vi "day4.vi"() -> ()   [LabVIEW 2025]
panel:
  out "Array 4":string[][](array[string])
  out "Array 3":i16[][](array[numeric])
  out "sum":i16
  out "size(s)":i32[](array[numeric])
  out "Array 2":i16[](array[numeric])
  out "x < y?":bool
  out "Array":string[][](array[string])
  out "subarray":string[][](array[string])
  out "appended array":string[][](array[string])
  in  "s":bool
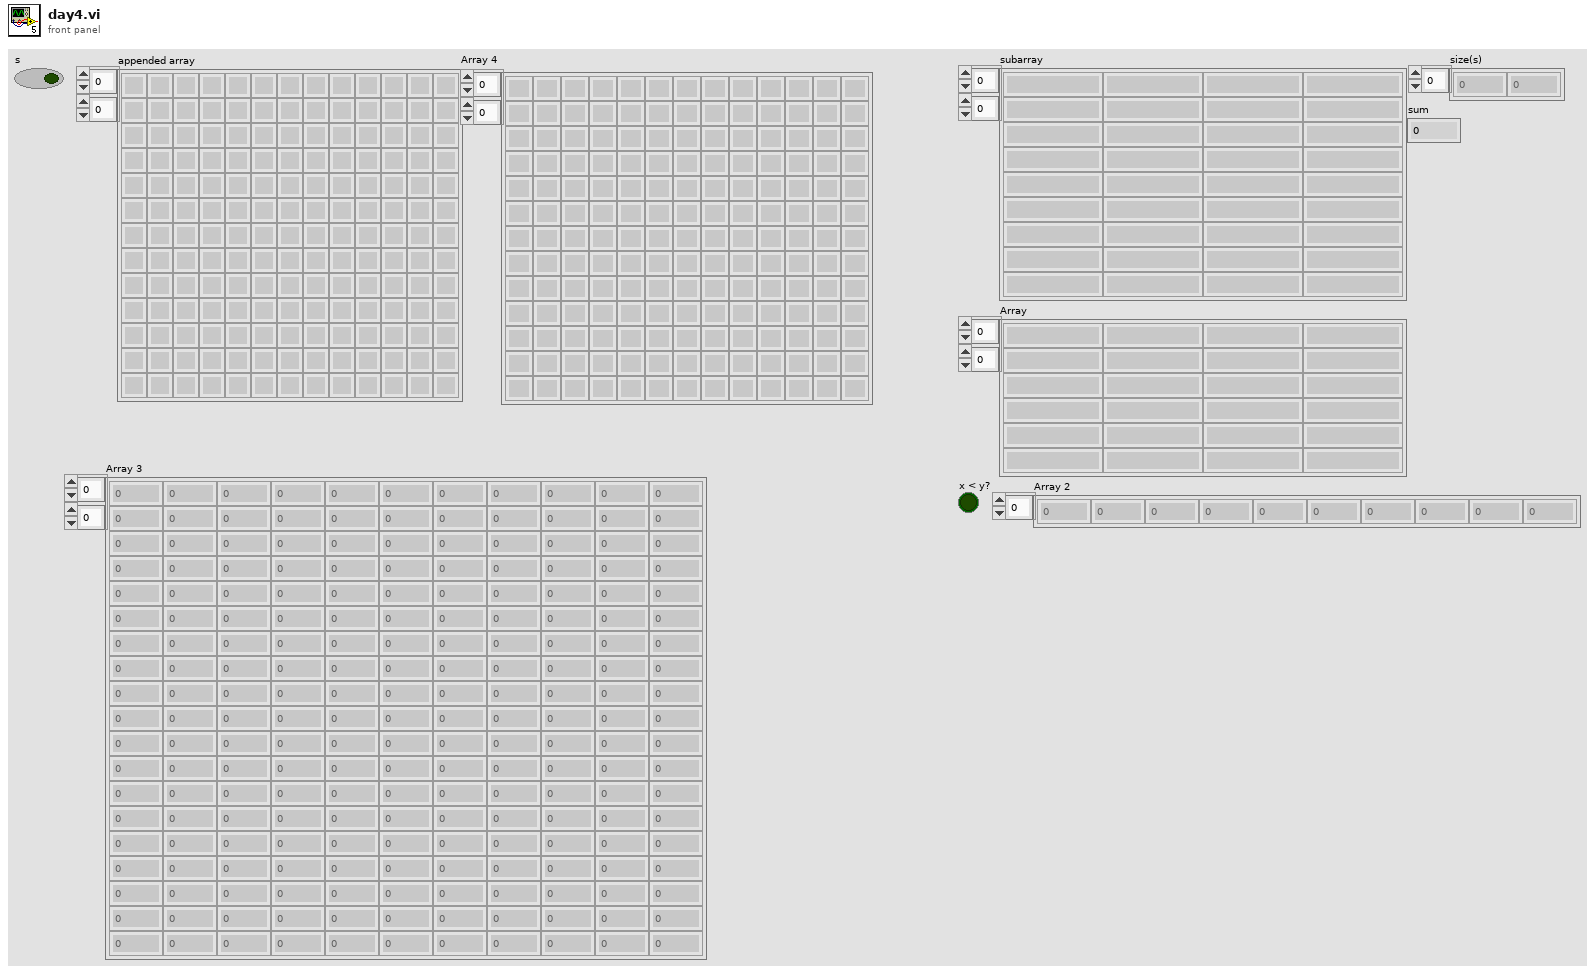
[diagram p1: front panel]
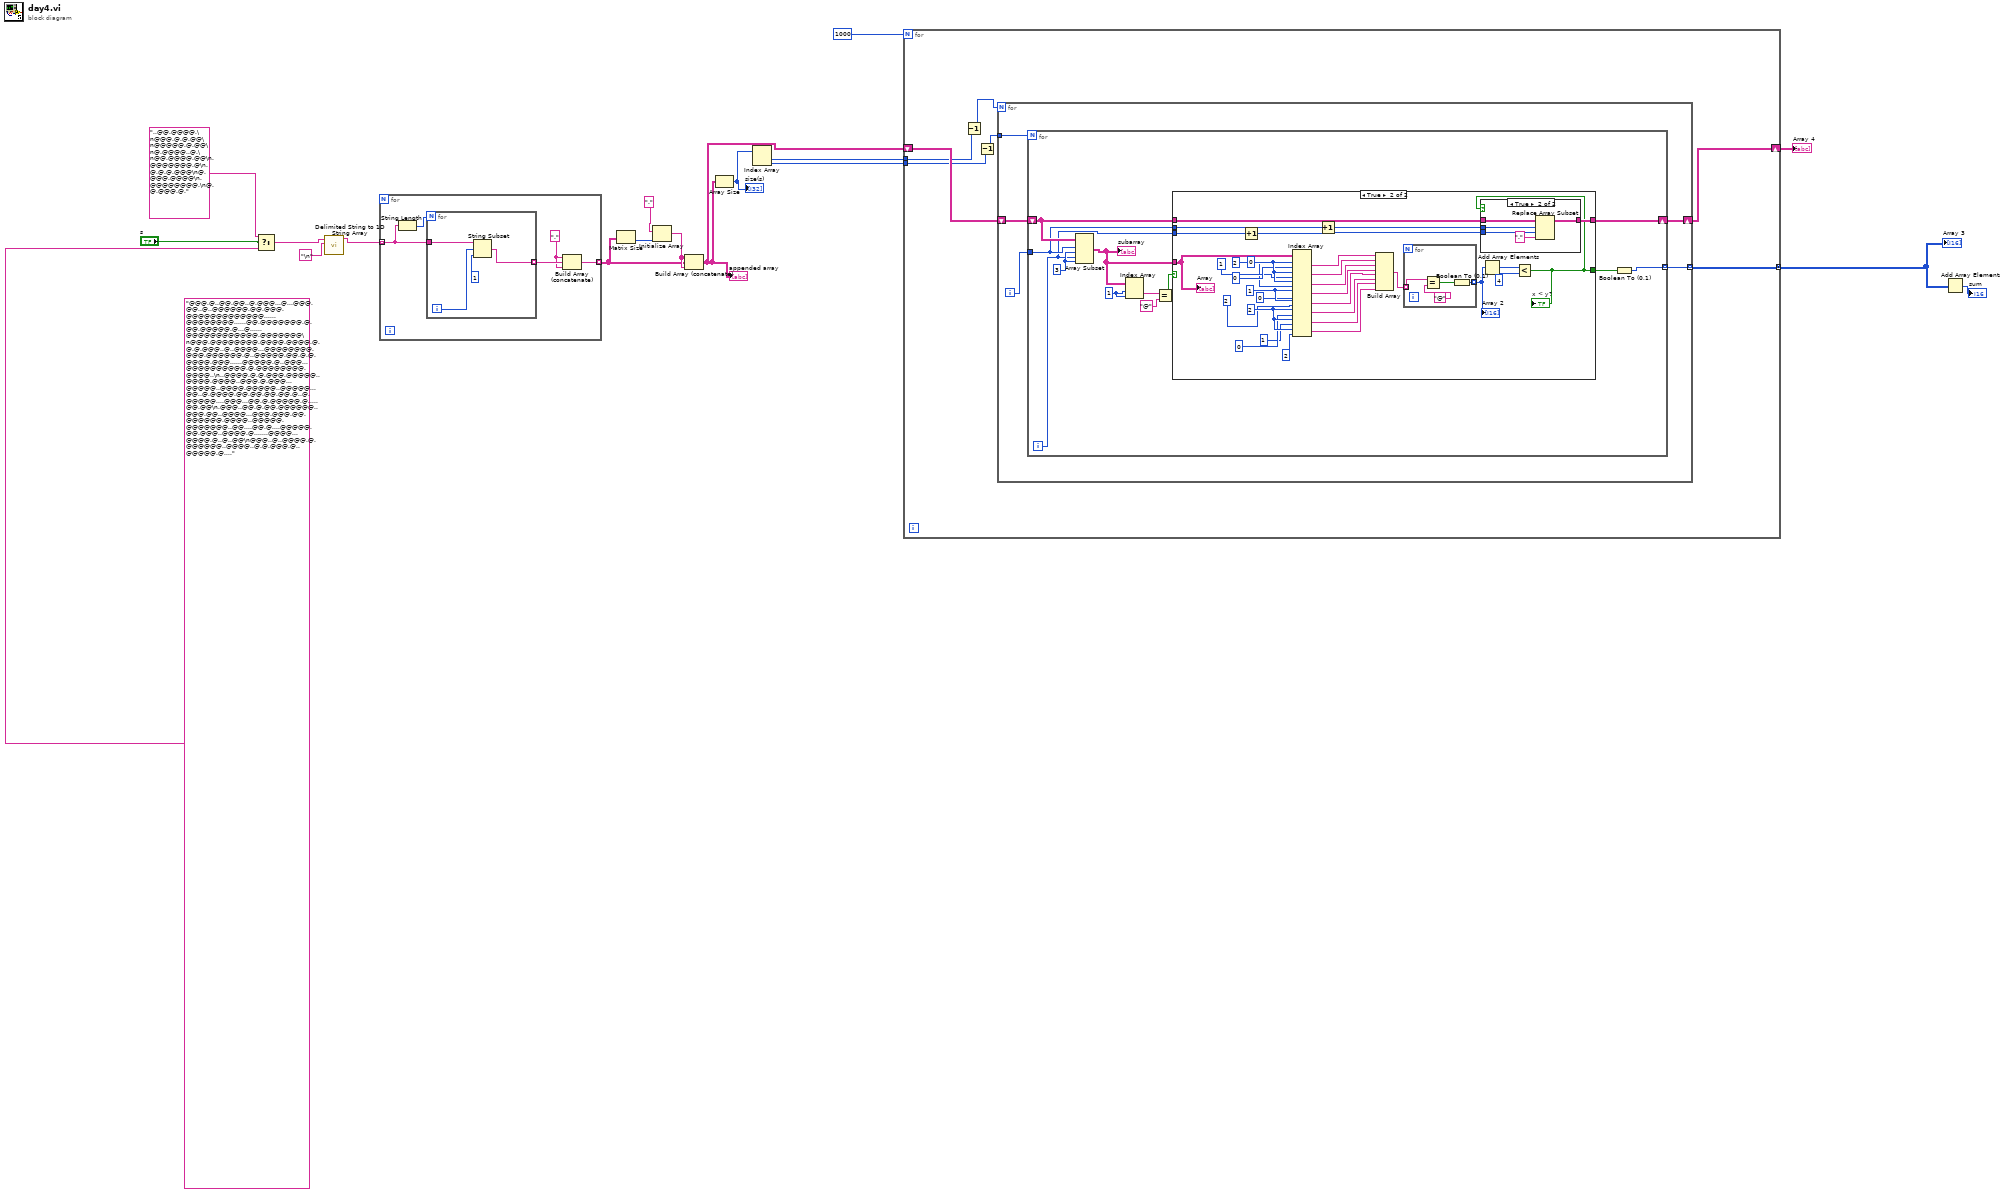
[diagram p0: block diagram]
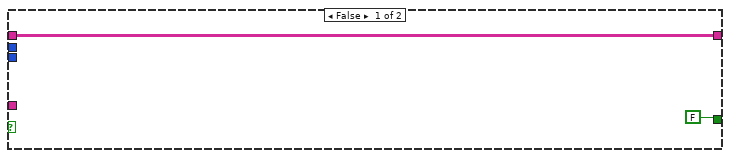
[diagram p2: hidden frame]
diagram:
  n1 = Select(t="..@@.@@@@.\n@@@.@.@.@@\n@@@@@.@.@@\n@.@@@@..@.\n@@.@@@@.@@\n.@@@@@@@.@\n.@.@.@.@@@\n@.@@@.@@@@\n.@@@@@@@@.\n@.@.@@@.@.", s="s", f="@@@.@..@@.@@..@.@@@...@...@@@.@@..@..@@@@@@.@@.@@@.@@@@@@@@@@@@@......@@@@@@@@......@@.@@@@@@@.@.@@.@@@@@.@...@......@@@@@@@@@@@@.@@@@@@@\n@@@.@@@@@@@@.@@@@.@@@@.@.@.@.@@@..@..@@@@...@@@@@@@@.@@@.@@@@@@.@..@@@@@.@@.@.@.@@@@.@@@......@@@@@.@..@@@...@@@@@@@@@@.@.@@@@@@@@.@@@@..\n..@@@@.@.@.@@@.@@@@@..@@@@.@@@@..@@@.@.@@@...@@@@@..@@@@.@@@@@..@@@@@...@@..@.@@@@.@@.@@.@@.@@.@..@.@@@@@....@@@...@@.@.@@@@@.@.....@@.@@\n.@@@..@@.@.@@.@@@@@@..@@@.@@..@@@@...@@@.@@@.@@.@@@@@@.@@@@..@@@@@.@@@@@@@..@@....@@.@....@@@@@.@@.@@@..@@@@.@.......@@@@...@@@@.@..@..@@\n@@@..@..@@@@.@.@@@@@@..@@@@..@.@.@@@.@..@@@@@.@...@..@..@...@....@@..@@@...@@@@@.@.@........@..@@.@.@@...@@@@@.@@@@..@.@@@@...@..@@.@@..@\n@.@@.@.@..@@@@.@.@@@...@@@..@.@.@@..@.@@@......@..@...@.@@.@@@.@@@.@@@@..@@.@.@@@@.@..@..@.@@..@@@@.@@@@@@@@@@@@..@@@@..@@.@.@@..@@..@..@\n.@...@@......@..@@@@@...@@@@@.@@@.@@@@@.@@..@@@@@@@.@@@@@@@@@.@.@..@@@@...@@.@...@@@@@.@@@@@...@.@.@.@@.@@.@.@@.@@@@.@@@@@@@@@.@.@.@...@.\n.@@@...@@@.@....@@@@@@@.@@@.@@@@.@@...@@.@@@@@@...@@@@@..@.@...@.@@..@@..@@@@@@.@@@@@@@@@@..@.@@..@..@.@@..@@.@@@@@@@@...@....@.@@@@@@@@@\n.@..@@@@@@@@.@@@.@@@@@@@.@@@@@.@.@.@@@@..@..@@@..@@@.@@@@.@@.@@@@@..@@@.....@@@.@.@@@@.@@.@.@@@@.@@...@.@@@.@@@@@@@@@..@.@..@@@@@@@.@@@@@\n.@.@@.@.@@@@@@@@@@@..@@@@@@....@@@.@.@.@@@.@@@@@@@@.@@@@@@@..@@..@@@..@@@...@.@@@@..@@@@..@@@@@@@@@@@@.@@.@@@@@@@@@@..@.@.@.@@.@@.@....@.\n@@.@@@@@..@.@.@@@@@@..@@@.@@.@.@@..@@@@.@@..@@@@@@@@.@@@@@@@.@@@@@@@.@@@@...@@@@.@@@@@@@.@@..@@.@.@@@@@.@@@@@@@.@@@@@@@@.@.@.@.@@@@@@@@.@\n..@@.@..@@.@..@.@.@.@@...@@@...@.........@@.@.@@@.@.@@.@.@@.@@@@@@@@.@.@.@@.@@.@@@@@@@@.@@..@@@@@.@@.@@@@@@.@.@.@@@.@.@.@.@@@.@@.@@...@@@\n.@@.@@@..@..@@@....@@@.@@@@@@@@..@@@@..@@.@@@@@..@@.@..@@@@@@@.@@@@@.@@@@.@@@@@@@@@@@.@..@@@..@@.@.@@....@@..@@.@@...@..@@@@@@@..@.@@@@@@\n.@@.@@@@@@.@@@@.@.@.@..@@@@.@..@@..@.@@@@@.@.@@@@@@@@@.@@@..@.@.@.@.@@@@@@@@@@@@...@@.@@@@@@@..@.@.@@@..@...@...@@@@.@@.@@@.@.@.@@@...@..\n@@.@..@@..@@..@.@@@.@@@@.@@@@@@@..@.@@.@@@.@.@.@@@@@@.@@@.@.@@@@@@.@@.@@@.@@@@@@@@@@@@@@@.@.@@@@@@..@@@@..@@.@@.@@@@@.@.@@@@@.@@@@.@@@@@.\n@@@@@.@.@@@.@@..@@.@.@@@@@.@@@..@@@@@@..@...@....@.@@..@@@@.@@@@.@..@@.@@.@@@@.@..@@.@@@@..@@@@.@.@@..@@@@.@.@.@.@@@.@@@@@@.@@@@.@...@@@@\n@@.@@@..@..@.@.@@@@@@@@@@@....@@@@@@@.@.@@@....@@.@@@@@@@@@@..@@.@@.@.@.@..@@.@.@.@...@@.@.@@@@.@@@@@@@@@@@...@.@..@.@..@@@.@@@.@..@@@@..\n.@..@@@..@@.@@.@..@@@@@@..@@@@.@@@@@@@@@@@@.@.@.@@@@@@.@@.@@@@.@@@.@..@@@@@.@@@@@.@.@.@@@@@@.@.@@.@.@.@@@@.@..@@@.@@.@@@.@@.@@@@..@...@@@\n@@....@@.@.@@....@.@@.@@@@@@@@@@@@@..@.@..@@@@.@@.@.@@.@.@@..@..@@@@@@@@@@@@@@@@@@..@.@@@@@@.@..@@@@@.@.....@@@..@...@@@@..@@@@.@@.@@.@@@\n.@...@@@.@@.@.@@.@@@@.@@@@....@@@@@.@@@@@@@@.@@.@@..@@@@.@@.@@@@@.@.@.@@.@.@@@@.@.@@.@@@@..@@@@@@.@@@@.@@.@@..@@@@....@@@@@@.@@.@@@@@@@.@\n.@@.@@@@@@@.@@@.@@.@..@@@.@@@@@@@.@@@@..@@@@@@...@@@..@..@@@@@@@.@@@@...@@@@@..@@@@@@..@@.@@.@@.@@@@@@@@@.@@@@@.@@...@@@@@@@.@@..@.@.@@@.\n@@@@@.@@.@@@.@@@@@@@@@@@@.@.@.@@@@.@@.@...@@@@@@...@@..@@@@.@@@@@@@.@.@@.@@@.@...@.@.@@.@@.@@..@@@@...@@.@@@@.@@@@@@@.@@@..@.@...@@@@@...\n..@@@@@@.@.....@.@..@@.@@@.@@@@.@@@@..@..@.@@....@@@@@.@..@@..@@..@.@@.@@@..@...@@..@@.@@@@@.....@@@@@@@@@@@@..@@@@@@@..@@@.@@.@@.....@@.\n@@@@@.@@.@@.@@.@@@@@@.@@.....@.@..@..@@@@@@.@@@.@@@@@@..@@..@@@.@@@@@.@@@...@..@@@...@@@@.@..@@@@@...@@..@.@@@..@.@@..@@@@.@.@.@@@...@.@@\n@@@@@@@@@@@..@@@@.@@@..@@.@.@@@@@@@.@@..@..@@@....@@@@@..@.@..@@@@@@...@@..@@@@@@@@@@@.@..@..@@@....@.@@@..@@@@..@@....@.@.@@@..@.@.....@\n@.@@.@....@..@@@@@@@@@@@.@........@.@@@@@@@@..@..@.@@.@.@@.@@@..@..@..@...@@@@@@@@.@..@@@...@@@@@@@@.....@@@..@@@.@@@.@@.@@..@.@@.@@@@@@.\n.@@@..@@@@..@@.@.@@@..@.@@.@@@@@@@@@@.@@...@@@@@@@@@...@@..@@.@@..@@@@@.@@@@..@.@..@.@@@.@@.@@@.@@@@.@@@@@@.@@.@@@.@@..@.@@@.@.@@@@@.@@@.\n@@@.@@.@@.@..@..@....@.@@@@@@@..@@.@@@..@@@@@..@@@@@...@...@@@@.@@@.@..@@@..@..@@@@@.@@.@@@@@@.@@@@@.@@@@..@..@@@.@@@@.@@...@..@.@..@@@.@\n@..@.@.@@@.@@@@.@.@@@.@.@@@@..@@@@.@@...@@@....@@..@@.@@@@@@@@.@.@@@@@..@@@@@@@@...@.@.@@@.@@.@...@@@@@.@@....@@.@@@@@@....@.@.@@@@.@.@@.\n@@@@@@..@@..@.@.@...@@@..@....@..@@..@@@@@@@@..@.@...@@@@@@@.@.@@.@@@.@...@@.@@@@@..@@@@@@..@@@@@.@@@.@@@@@@.@@...@@@@@.@.@.@@@@..@.@@..@\n@...@@@@@@@@@@@@.@@@@@@@..@..@.@@@@@..@@@..@@...@..@@.@.@.@@@.......@@@@@....@...@@@@@@@@@@@.@.@.@.@@@@@@.@@@.@@....@@@.@....@@@@@@@@.@@.\n@@.@@@.@@.@.@@@@.@.@.@@@.@.@@@@..@.@@@@@@@@@.@.@@@@.@@@..@...@@@.@.@.@.@@@@@@.@@@@@.@@@..@@@@.@.@@@@@@.@@@@@.@@..@@@@@@@@@@.@..@@@@@@@@@@\n@@.@..@@@@@.@@@@.@@@@@@@@@@@@...@@@@@.@..@..@.@@@@@@@@..@.@@@@@..@.@@@@.@..@@..@@@@@@@@@@..@@@.@.@@@@@@.@@@@.@@@@@@@@@@@@@.@@@@..@@@@@@@@\n.@.@@@@..@.@.@...@@@@.@..@@@@@@@@@...@@@..@.@@@..@@@@@@@@@...@@@@@@.@@@.@@.@@@@@..@@..@@....@@@@@@@@.@@@@.@@..@@@@@@.@.@@@@@.@@@@@.@@@@@.\n.@@@@@@@@@..@..@@@@.@.@.@@@@.@@@...@@.....@.@.@@@@@@@@@@@@@@@@.@.@..@@.@.@@@..@@..@@@@@@@.@@.@@@.@@@@@..@@.@@@@@@@@@@@@..@@@@.@.@.@.@@@@@\n@@.....@.@@@@@@.@@.@@@@@@@@@@@@.@@@@@@.@@@@@@@@...@@..@@.@@.@@@@@@@.@@@.@.@@@...@@@@@@@@.@@@@@@.@@@@.@@@@@@@@.@@..@..@..@@@....@.@@@@.@@.\n@....@..@.@..@.@@@@@@.@.@.@@@@..@.@@@...@@@.@..@.@@@@...@@@@@@@.@.@.@.@@@@@@@@@@@..@.@@..@@.@@@@@@@@...@@@.@@..@.....@@@@@@@@@@..@@.@@.@@\n..@@@...@.@@.@@@.@@@...@..@@@@@.@..@@.@.@@@.@@@.@@..@@@@@@@@@@@@@.@@@@@..@.@.@@@@@@..@@@@..@@@...@.@@@@....@...@@..@@@..@@@@@..@..@.@@...\n.@@@@@@@@.@.@@.@@.@@@@@.@@.@........@@..@@@.@.@@..@@..@@@@.@@@@@.@@.@@@@@@@.@@@.@@@..@@....@@...@@@.@.@.@@@@@@@@.@@@...@@@@@@@@@@.@..@@..\n@.@@.@.@@@@.@.@.@@@@@..@.@.@...@@@.@.@.@.@@@@@@@.@.@@.@@@.@@@@@.@@@@@@.@.@@..@@@..@.@@.@@..@.@@@@@@@@@@.@....@@@.@@@@@@@@@@@@@@@...@@@@..\n@@.@@@..@.@@...@@.@@@@.@@@@@.@.@@.@@@@@@@@@...@@@@@.@@@@@@..@.@@..@@@.@.@@@..@@.....@.@@.@.@.@..@..@@@.@.@@.@@@@@@@.@.@@....@@.@@@@...@@@\n@.@@.@@@@@..@@@@.@..@..@@.@.@.@...@@.........@@.@.@@@@.@@..@@.@@.@@@.@.@.@@.@@.@@..@.@@.@.@@@@@@@@@@@..@.@@@.@@.@@@@@@@.@.@@...@..@@@...@\n@.@@@...@@.@@.@@@@.@@..@@@.@@.@@......@@.@@@..@@.@@..@@@@@.@.@.@@....@..@@@..@@.@@.@@@@@@@.@@@@@@@@...@@@@@@@@@@@@@@@...@...@..@@.@.@@@@@\n@@@@.@@.@@@@@@@@@.@.@@....@...@@.@..@.@.....@@@.@@....@@..@@..@.@.@@@@....@.@@@@@@.@@..@@.@@@.@@@.@@@@@@@@@@@..@.@@..@.@.@@@@@@.@@@@@@.@@\n...@@..@..@@@..@.@@@@@@@.@.@@@.@.@@@.@.@@@.@@.@@@@@..@@.@...@@@..@.@@@@@@@.@.@@@.@@@@@.@@@@@@@@.@@.@.@@@@@.@..@.@@@@@@@@@@.@@...@.@...@@.\n.@@@@@@@@@@..@@@@.@@.@.@@@.@@.@@..@@@.@@@@@.@.@@@..@@@@@@@.@@@@@..@@@@@.@@.@@@..@@@@@.@@@.@..@..@...@.@.@.@@.@@.@@@@@@@.@@@@@.@@.@@@@..@@\n@..@.@.@@..@.@@@@@.@.@@.@..@@@.@@@@..@..@@@@@..@@..@@@@..@.@@.@@.@@@@@@@@@@@@@@......@...@.@@@@.@..@.@.@@...@@@@@@@.@.@@.@@.@@@....@.@@@@\n@@@@@@@@@@.@@@..@@.@@@.@@.@..@@.@@.@@@@@@...@..@.@....@.@@.@@@@@@.@@.@@@.@@.@@@@@......@@.@@..@@@.@.....@@@@@@@@.@@..@@.@.@.@@..@@.@....@\n@@.@@@..@@@.@@@@@@@@@@...@@.@.@.@@.@@.@.@....@@@.@@..@....@.@@.@..@@@.@@@.@..@.@..@..@@@@@@@@@.@.@.@.@...@@@@.@.@@@.@...@@@@@@..@@...@@@@\n@@@@.@@.@@@.@@@@@@@@@@@...@@.@@..@.@@@...@@.@.@.@@@@@@.@@@@..@@@@..@@..@.@.@@@@@.@.@@@@.@@@.@@@.@.@@@..@@.@@..@.@@@@@@@.@@@..@@@@.@.@@@@@\n@...@@.@@@@@@.@.@@@@@@@@@@@@@@@@@@..@@..@@...@@.@.@@@@.@@.@@@@@@@.@.@.@@.@@.@..@.@@@@..@@@...@@.@.@@..@@@....@@.@..@...@.@@@.@@@@@@@...@@\n@@..@..@.@.@@@@.@@@..@.@@@@@@@@.@@@.@@@.@@@.@@..@@.@@@@.@..@.@..@...@@.@@@@...@@@@@..@@@..@...@.@@.@@@.@.@@@.@.@....@..@.@@@@@@@@.@@.@@@@\n@@@@@@..@@@....@@.@.@...@@@@@.@..@@@@@@..@...@@.@@@@@@.@.@@.@@@@.@.@.@@@@@@.@.@@@@@@@@.@...@@@@@@.@.....@@...@@...@@@@@@@.@@@@@@@@.@.@@..\n@@@@@@@@...@@@@..@..@..@@@..@@.@@@@@@.@@@..@@@@.@@.@..@..@.@@.....@.@@..@@@....@@@@@@.@@@@@@@@@@@@..@.@@@@@@@@....@.@@@.@@@@@@@@@@@..@.@.\n@@@@@.@..@.@@.@@@@..@.....@.@@@.@.@.@@@.@@@@@..@@.@@@@@@..@@.@.@@@...@@.@.@@..@.@.@@..@.@.@@@@@.@@..@..@@@...@@@.@@@@@@@@@...@@@.@@..@@@@\n..@@...@@@@@@@@@@.@.@.@..@@.@@@@@@@@....@@@.@..@@@@.@@@@@.@.@@@.@@.@@.@@@@@@@@@..@@.@@@@@@.@@@@@@@..@@@...@@.@@@@@@@@.@.@@@@@@.@@@@......\n@@...@...@@@.@..@@@.@@@@@@@@@@@@@..@.@@.@@@@@@@@@@.@@.@@.@@.@@@@.@.@@..@@@@.@@.@@.@...@.@......@@.@..@.@@@@@@.@@@@@@....@.@....@..@@@@..@\n@.@@@@@@@@@.@.@@@@@@@@@@@@..@.@@@@.@@.@@.@.@@@...@@@.@@@.@@@@..@@@@@@@@..@@.@@..@.@@.@@@.@.@@@@.@@@.@@@@@@.@@.@@.@@@...@@@@@@.@@@@.@@@.@.\n@@@.@@@@@..@@@@@@.@.@@@@.@@...@@@@@.@@@@.@.@.@.@@.@..@@..@@@@@@...@@@@.@..@@@..@@.@@@.@@@@@@@@.@@@@@@.@@.@.@@@@@@@@@@@.@.@@..@@@@.@.@.@..\n...@@@..@..@@..@@@@@@@..@@.@@@...@@.@@@@@@.@@@@@..@@@.@@@@@@@@@.@@@@@@.@.@.@@@@@..@@@@@@.@@.@@@@.@.@@@@@@@@..@@@@@@.@.@.@@.@...@@@@@...@.\n.@@@....@.@.@.@@@@.@@@@@@@.@@@@.@.@@@@@@.@@@@.@@@@..@@..@..@@.@...@@@@@.@@@@@@@@.@@@@@@.@@@@@.@@@@@@@..@.@@@@@..@.@@@@.@@@@..@@@@@.@.@.@.\n..@..@.@..@@@@@.@..@.@.@@@@@.@@@@..@.@@@@@...@.@@.@@@@.@@@@.@.@@..@..@....@@.@.@@..@.@@@@.@.@@.@....@.@@.@@..@..@@..@@@@@@@.@@.@.@@@@....\n@..@.@...@@.@@@@.@@..@@.@@..@@.@@@@@@@.@@@@@@@.@...@..@@@@..@@@@.@...@..@@@@.@.@@@@.@.@...@.@.....@.@@.@@@@.@@.@@@@@@@@@@.@..@@@.@.@@@@..\n@@@@.@@@@..@.@...@@@@.@.@@.@.@..@.@@@@@.@@.@@@.@@.@@....@.@@@@...@@@..@@@..@@@@@@@@@@@@.@@@..@@@@.@@@@@@@@.@.@@@.@..@@.@.@@@.@@@@..@@.@@@\n...@.@.@.@@@@@@@@.@@@@@@.@@.@@.@.@...@...@@@@@..@.@@@...@@@.@@@@@.@@@@@@@@@@@.@..@@@..@@.@@@@@@@@...@@@.@@..@@@@.@@@@.@@..@@@@@.@@@@@@..@\n@@..@@@@.@..@.@.@@@....@@.@@@@..@...@...@.@@..@@....@@.@@@@.@@@..@...@@@.@@@.@@.@..@@@..@..@@@@@@..@@.@@@@@@@@@@@.@@.@@@@@...@@@@.@@.@@@.\n@@@@..@.@.@@..@@@@.@@@@.@@@@@@.@..@@@.@@.....@.@@.@@.@.@@@@@.@@@@..@.@@..@...@.@@@@@@..@.@@..@..@@@@@.@@@@.@...@@..@..@@.@@@@.@.@@@@@.@..\n@.@..@@@..@@.@@@@@.@@@...@@@@@@.@@@@.@.@@@@@@@@@@@.@@@@.@@@@@@.@@@@@....@@..@@@@@@@...@.@..@@@.@.@..@@@..@@....@..@@@@@.@@@@@@.@@@@.@@@@.\n@@@....@@@.@@@.@.@@...@@@..@@.@.@@.@@@.@@@@@@@@@.@@..@@..@@@@..@@@.@.@@..@..@@.@.@@@..@@@@@@@.@@.@.@@@@@.@@@@.@@@.@@@.@.@@.@@@.@@@.@@@..@\n@.@@.@@@@@@@.@@..@@@@@@..@@@@@@@@.@@@@.@@@..@@.@@@@@@@@@@@.@@...@@@@.@..@@@.@@@@@@@@@@@@.@@@@@@@@.@.@@@@@@.@@.@@@@@@@@.@....@.@@@@.@@.@..\n@.@@..@@@@@@@.@@@@@@.@..@@.@..@.@@@.@.@@@..@@@@@@@@@@@@@..@@@@.@@.@@@@.@@@@.@..@.@@.@.@@.@@@..@.@@@@@.@@.@@.@@.@@@.@@.@@@@@..@@..@.@.@@@.\n.@.@..@.@@@@@@@@@@@@@@..@@@@..@@@.@@@@@.@@@.@@@@@@.@..@@@.@.@@@@@@.@.@@.@.@..@.@@@@@@..@..@.@@@@@@@@@.@@.@@....@.@@.@@@.@@@.@@.@@@@.@@@@@\n...@@@.@@@.@.@.@@.@@@@@@@.@..@.@@@@.@.@..@@@@.@@..@@.@@@@@@@@.@@@.@@@@@...@.@@.@..@.@@@@@@@@.@.@@.@.@.@@@.@@@@@@.@...@..@.@@.@..@@@@@.@@@\n@...@.@..@...@@@.@@...@.@.@.@@@.@.@@@@.@@.@@@@..@@.@@@@..@....@..@@...@.@@@@@@@@.@.@@@@@...@@@...@@@@@.@.@@..@@..@@@.@.@@@@@@@@.@@@@.@@@.\n.@@@..@@.@@@@.@.@..@@@@.@.@..@@.@.@@.@@.@@@@@@.@..@@..@@.@@@@..@@@@@@@@..@@@..@@@@..@@@@@@@@@@.@.@@@..@@@@...@@@@@.@@@.@@@@@@@@....@@.@@.\n@@@.@@..@@@.@.@.@.@@..@@@..@.@@@.@@...@@.@@.@@@@.@@@@@@.....@@@@@@.@@.@...@@@.@@@.@.@@@@.@@.@..@@.@@.@@@..@..@@.@@@..@.@@@@.@.@@@@..@.@@@\n@@@.@@@@@@@.@@@@@.@.@@@@@@.@@....@@@.@.@@@@..@@.@@@@.@@...@.@@.@@@.@.@...@@@.@@.@@.@.@@.@....@@.@@@..@@@@..@@@@@.@@.@@@@@@@@@@@..@@@@@@@@\n@..@.@@@@.@@@.@..@..@@@.@@@@@@@.@.@...@..@.@@@..@.@@@.@@@@@.@@@@@@@.@@@.@@....@@@.@@..@.@@@.@.@@.@.@.@@@.@.@.@@..@@@@.@@.@@.@@@@@@@..@.@.\n@.@@@.@@.@@@@..@.@@@....@@@.@@@@.....@@@.@@...@....@.@.@@...@@@...@.@@@..@@@@.@.@@@@@@@@.@@@@.@.@..@@.@@@.@..@@.@@.@@.@@@@...@.@@@@...@@@\n.@@@@@@@@@@@@@.@@@@.@@@@..@..@..@@@.@.@@.@@@..@@@..@@.@@.@@@@@@.@....@.@@@@@@@@@@.@@...@..@@..@@.@.@@@.@@@@@.@@..@@@..@@.@@@.@.@@@...@..@\n@@@@@@.@...@@@...@.@..@@@@.@..@....@@@.@.@...@@.@@@..@.@@...@.@@@@..@@.@@@.@@@.@@@@@@@@@@@@@..@.@@.@@@..@@@@@..@@.@@.@@@@@@@@..@.@@@@.@@@\n@@@@.@@...@@@@@..@.@@@@..@@.@.@@@@@@..@@@.@.@.@@@@..@@@@@...@@@.@@@..@.@.@@.@.@@.@@...@.@...@..@@@@@@@@@..@@@....@@.@.@@@@.@.@.@@..@@@@@.\n.@@@.@@@.@@.@@@.@@..@@@.@.@..@.@.@.@@@@@@@.@.@@..@.@..@...@.@@@.@.@@@@..@@@..@@@.@@@@@@@...@@...@.@@..@@@@@@@@@.@@@@@@@@@@@.@@@@@.@.@.@@@\n@.@@@@.@..@@@@.@@@@@.@@@@@@.@@@@.@.@@.@.@.@@@@@@@...@..@@@@@@@@@@.@.@@@..@.....@@@@...@....@@@@@@.@@@@@@@.@.@@.@.@....@@@@...@@@@..@.@@@.\n@@@@@.@.@@@..@@.@.@@..@@@.@@@@@.@...@..@@@.@@@@.@@..@@.@..@...@.@@@.@.@@@.@@.@.@..@.@..@.@@@..@.@.@@@@.@..@@@.@@@@.@.@..@@@.@@@.@@@@@.@@@\n@..@@@@.@.@.@@@@@@@@...@@@@@@..@@@..@@.@@..@@@@@..@@@@@...@.@.@@@@..@@@@@..@.@.@@@@.@.@@@.@@@..@..@@@.@@@..@.@.@@@@@@@@@@.@@.@...@@@@@@@@\n@.@@.@@.@..@.@@@.@@.@.@@.@.@..@@@@.@@.@@@@.@@@@@@@.@@@..@.@@@@@..@.@@@@@@...@@@.....@.@.@@@@@@@.@@.@.@.@@@...@@@@@@@..@@@@.@@@.@@@@.@@@@.\n@@@@.@..@.@@@.....@@@.@.@@.@@@@@.@@@.@@@@...@@.@.@.@@@@..@.@...@@@@@@@@@..@@.@@@@.@@.@@@@.@@..@@@..@.@@@@...@@@@.@..@@@@@@.@@.@..@@@.@.@.\n@@@.@@@@@.@@.@@.@@@@@@@@.@@..@.@@...@@.@@..@.@@@@@@.@..@.@@@..@@@.@@.@@.@....@@......@@.@@@..@@@..@@.@@@...@@@@@@@.@....@@@@.@@@@..@.@@..\n@@@@@@.@....@@.@@.@@@...@@.@.@@@.@.@@@@@.@@@.@..@@@@@@.@..@@@.@@@.@..@@.@@@@@@..@.@@@.@@@.@.@@@..@.@@...@@@.@@.@@@@@@@@.@@@@.@..@@@.@..@@\n@@.@.@.@@@@@@@.@@.@@@..@@.....@.@@.@@@.@@@.@@@@@@@@@@.@.@.@@@.@@.@.@..@@@@@@@@.@..@..@@@@@@@@@.@@@@@@..@.@..@..@@...@@@@.@.@@@..@@@@.@.@@\n.@@@@@.@.@@@@@@@@@@@@@.@@..@@@@@@..@@.@@@@@@@@.@@...@@@@@@.@.@.@@@..@@...@@.@.@@@@@@@@@.@@...@@@@@.@@@@@..@@@@@@.@@@...@@@.@@@@@@@@@@....\n@@@@@@.@.@.@.@@.@@.@@@..@..@@.@@..@@@@.@@.@.@.@@.@@@@@@@@..@@@.@.@.@.@@@@.@......@.@.@@@@@@@..@@@@@@.@..@@.@.@.@@..@..@@@.@@@@@@.@@@@.@@@\n....@@@@@@@@@@@@@@@.@@..@@.@@@@@..@...@.@@...@@..@@@@@@@@@@@@@.@.@.@@@.@.@@.@.@@@.@@@@@@@.@@@@.@@@@@.@@@@@@@..@@@@@...@...@@.@@@@@@..@@@.\n@@@.@@@.@.@@@@@.@@@@@.@@@..@@..@@@@@..@@@@.@@...@@.@..@..@@@@....@.@.@@.@@@@.@....@@@.@@..@@..@@@@.@@@@@..@@@...@@@.@@@@@@@@@@@@.@..@@@.@\n..@.@.@@@@..@@@@..@@@@.@@@.@..@@.@@@@@@.@@.@.@.@..@@@@@.@@@@..@.@..@.@@@@@.@.....@@@...@.@@@@..@..@..@.@@.@.@@@.....@@.@@.@@...@@...@@@@.\n@.@@@..@@....@..@@.@@.@.@@.@.@.@@@.@@@@@....@...@@@.@@@.@.@@.@.@@@@@@.@@@.@@.@@@@@@..@@@@.@..@.@@@.@.@@@...@.@.@..@@@@.@@@@@@.@.@@...@@@@\n@@.@....@@@@@..@@@..@.@@.@@@..@@@@@@@@@@@@@@@....@@.@@@@.@@@@.@.@.@@.@.@.@@@@@@@@.@@.@@@@@@@..@.@@@@@@@.@...@@@@@@@....@@@..@....@.@@@.@@\n@.@.@@@@@@@@@.@@@@@@.@...@@@.@@@..@@@@.@.@@.@@@.@.@@.@@@@@.@@@.@@@@.@@..@@.@.@@.@@.@@@.@.@@@@..@@@.@@@.@..@@@@@.@@..@@..@@...@@@@@@@@@@.@\n.@@@@@@@@@.@..@@.@@@@..@..@@@@@.@@...@.@@.@.@@@@@@@@@.@@@@....@@.@@@@@...@...@.@@@@@.@@@@@@.@..@@..@.@@@@@.@@@@.@@@@.@@.@@@.@@.@...@@.@@.\n..@@@@@@@.@@@@@@@@@@@@@@..@@@.@@@@@@..@@@.@@.@@@@@@@@@@@.@.@@..@@@@@.@@@.@.@@@@..@...@@.@@@@.@@@@.@@@@@..@.@@@@.@@.@.@.@.@@@.@@.@@@..@@@.\n@@@@.@@@@.@@.@@@@@@@.@.@@@@@@.@.@.@.@@..@@....@.@@@@@.@..@.@@...@.@@@@@@@.@.@@@.@.@@.@@...@@@.@..@@@@@@...@@..@@@.....@.@.@@@@@@...@@@@@@\n@..@..@@.@@@..@@.@@.@.@@@...@@.@@@.@@.@@@.@...@@@@.@.@@.@@@.@..@@@@.@@@..@@..@@@@.@.@..@..@@.@.@@@.@...@@@.@@@@@@@.@@@.@.@..@..@.@@@@@.@.\n@@@@..@@.@@@@.@@@@...@.@@@@@@@.@.@@.@@@..@@.@@@@@@@@@@@.@@@..@.@@@.@@@@..@@@@.@@@@.@..@.@@@..@..@@.@@@@@@.@..@@@@@@@...@.@@.@...@.@.@@..@\n@@.@@..@..@@@@@@@@@@@@@@..@@@@@@@.@@@@@...@@@..@@.@@..@.@@@@@@@@..@@.@.@@.@@@@@...@@@@..@@@@@@@@@@@@.@@@..@..@@@@.@@@@@@.@@@@@@@.@...@@@@\n@@@@@.@@.@@...@.@.@@@@@@@.@@@....@@@@@@@..@@..@..@@@@@..@@@.@@@@@@@@@.@@.@.@@@.@@...@@@.@@@.@@.@@@.@..@@@@@@.@@@@@@@@@@@...@.@@@@@@.@@@@.\n.@@@@@@.@@@@..@..@@..@@@.@@@@...@@@@.@..@@.@@@@.@.@.....@..@.@@...@@@@.@.@..@@@@@@@..@@@@@@@@@@@@@.@..@@@@.@.@..@@@.@@@@@@..@.@@..@.@@.@.\n@@@.@@@@@...@@@.@@@@@.@@@@@@...@@.@@.@@.@@@@@@@@.@@@@@@.@@@@..@.@@.@@@@@@.@.@@.@@@.@@@@.@@@@@@@@.@@@@@@@@.@@.@@@.@.@@@@@@@.@.......@.@..@\n@@@@@@.@..@...@..@..@@@..@@@@.@@..@@.@@@..@@.@@@@.@@@@@...@.@@@.@@@@..@...@@@...@.@@@.@@@@@@.....@@@@..@.@@@.@@@@@@@.@@@.@.@.@.@@....@..@\n@@@..@@@.@..@@@@....@.@@@.@@@@.@@@@@@@.@@@.@@@.@@.@@@.@@@@.@@@@.@@@@.@@..@@@@@@@...@@@.@@@@@@@.@@.@.@@@@@@@@@@@@@@@@@@@.@.@@@@.@@@.@.@@@.\n@..@@@@@@@@@@@@@.@.@.@@@@..@.@@@@@@.@@@@..@..@@@@.@@..@@.@@@@@@.@@@@.@.@@@@@.@@@@@@.@@.@@...@@@@..@@@@@@@@@.@@@.@@@@@@@@@@.@.@@@@@@@@.@@@\n@@....@..@..@...@@@@.@...@@@.@@.@@@...@..@.@@..@@@.@@@@@@...@.@@@.@@@@@.@@@@...@@@@.@@@@.@.@@.@@@@@@@.@.@..@@@@@@@@@@..@.@@@@.@..@@@@@@.@\n.@.@@@@@@@@..@@.@@@.@.@.....@@@@.@@@@@@..@...@@@@.@.@@....@.@@@@@.@.@@@.@..@.@@@@@@@@@.@@@@@@@@@@@@.@.@@.@...@@@@.@.@..@.@@@@.@..@@.@@@@.\n@@@@@.@.@@@@@@...@@@@@@@@@@@...@...@.@...@..@@.@.@@@.@.@..@@@@@@@@.@.@@@@@.@@@@@@@@@.@....@@@@@@.@@@@@@@.@@@@.@@@@@@@@@...@..@@...@@.@@@@\n@..@.@.@.@@@..@@@..@@@@@@.@@@@@@@@@.@.@.@.@@@......@..@@@@.@@@.@@.@@.@....@.@@@...@.@@@.@@@.@..@...@@@@@@@@@@@@@.@.@@@.@@@@@@@@@.@@@@@@@@\n..@@.@@@@@@@@@..@@...@..@@@@.@@.@@@@@@.@@.@.@..@@@@@@@@...@@@@@.@@.@@@@@.@.@@@.@@@@.@.@.@..@@@@@@.@@@@@@.@.@@@@....@@..@..@@..@@..@@@.@@@\n@@@.@@@@@@@.@@@@@.@@.@.@@.@@@@..@@.@@@@@@...@@@@@@..@.@@@.@@.@@@@@@@@@@@@@....@@@@..@@@.@@@@@@@@@.@.@@@@@.@@@@@@@@.@@@@.@..@@.@.@.@.@@@@.\n@.@@@@@@@@@.@@.@@.@@@@@..@.@@@.@..@....@@@@.@.@@@@.@@.@.@@@..@@..@@.@@@@@@@@@@@@..@.@@@@.@....@@.@@@@@@.@@@@@@.@.@@@@@.@.@@.@@@@.@@..@.@.\n@.....@.@@@.@.@...@.@.@@@@@@@@@@@@..@.@@@@@@@@@@@@.@@@..@@@..@@@.@@@@@.@@@@@@@@@@@@@..@@@@.@..@@@@..@@..@@@@@@@@@@..@@@@@..@@@@.@@@@@.@@.\n.@@@@..@.@@@@@...@@.@@@.@@@@@@@@@@...@..@@.@.@..@@@@@@@...@@@@@@@.@.@....@.@.@@@.@@.@@@@.@@.@.@@@@@@.@...@@@@.@@@@.@.@@@.@@.@@.@@@@@.@@@@\n.@@@.@@@@@@@@@.@@@@..@@@.@..@@.@@@.@@@@@..@@@..@..@.@.@@@....@@@..@.@.@@.@@.@..@@.@@@@.@@@@@@.@...@.@@@@@.@.@..@@@..@.@...@.@@....@@@@@@@\n@@.@.@@@@@.@.@..@..@@@@.@@.@@..@@@.@@.@@.@@@.@.@@@...@..@.@@..@@@....@..@@@.@@@@@@@@@@@@@@...@.@@..@@@.@@...@@.@@@..@@@@@@@......@.@@@@@@\n@.@@@..@@.@.@@@.@.@..@.@...@@.@@..@@@@@..@@....@@@@@@.@.@.@@@.@@@@@@@@@@@@@@.@@.@@@@@@.@.@@@...@@@@.@@..@...@.@@.@@@@@.@@@.@@@@@@@.@@..@@\n.@.@@.@@@.@.@@@@@@..@.@.@@.@@@.@@@@@...@@@@@@@@.@@@....@...@@.@@@@.@...@@@.@.@@@@.@@@@.@@@@@@.....@...@.@@@@@..@..@.@.@...@..@@..@.@@@@@.\n@@@@.@@.@@@@@@@@@..@...@@@@@@@@..@@@.@@@@@@@..@@@.@@@@@@@@@..@@@@@.@@@@..@@@@@@@@.@@@@@@@@@@@@@@@@@@@@@@.@@..@@@@@@@@@@@@.@@@@@.@@@@@.@.@\n@@.@@@@@.@@@@..@.@@..@.@@@@.@..@@@@.@@@@@.@@@.@...@@.@@@@@..@@@.....@.@@@@.@.@@@@@@.@@..@..@@@@.@@@.@@..@.@@.@@...@.@@@@.@@@@@...@@.@@@.@\n@@@@@@.@.@.@@@.@@.@@..@@.@@.@@@..@.@.@..@@.@@@@@@@.@.@@..@@@@@@@@@.@.@@..@@@@@@@@.@.@.@@@@@@@@@.@@...@@@.@@@@....@@.@@.@@..@@@.@.@.@@@.@.\n@@@@@...@@..@.@@.@.@.@@...@@..@@@@@@@@@.@@@.@@@.@@...@@@@.@@@.@@@@.@@..@@@@...@.@@@@.@.@@......@@@@@@@..@@@.@@@..@..@@@@@.@@@.@@.@@....@@\n@..@@.@@@@@@@@....@.@.@@@@@@....@@@@.@.@@@.@.@@@@@@@.@@@@@@@..@@.@@@.@..@@@@@@.@.@..@@@.@@.@.@@@@@@@....@@.@.@@.@.@.@@@.@@@...@@@@@.@@@..\n.@@@@..@@@@.@.@@.@@@@....@@@..@.@.@.@.@@@@@@@@.@.@.@@@.@@.@@..@@.@@@@.@..@@.@@..@@@.@.@.@..@@...@.@@@@@.@..@@@@@.@...@.@@@@@@@@@@.@.@@..@\n.@...@.@@@...@@@.@@@.@.@@@@@@.@.@@@@@...@@@@@@@@@@@..@@.@@@@@@...@@.@.@@@.@.@@@.@@@..@@@@.@@.@.@@@@.@@@.@@@@@@@@@@@@.@@@@@@@@@@@.@@@@@.@@\n@.@@@.@@@@@@.@@.@..@.@@.@@.@@..@.@@...@@@@@@@@.@@@..@.@.@.@@@.@@.@@@.@.@@.@@@@@....@@@.@@.@@.@@..@@@..@@@@@@.@@@@@@@@@@@@.@@.@@@@@@@@@.@.\n@@.@@@@@@.@.@@...@@.@@@@..@.@.@@.@@@.@...@@@@..@@.@@.@@.@.@@@@..@.@@@@.@@@..@@.@.@.@@@@@@@@@......@@.@@@@@@...@.@..@.@@@@@..@..@.@@.@@..@\n@@@@@@..@@.@@@@..@@@.@@@@@..@@@.@@@@@@@.@@@@..@@@@.@@@.@.@@@@@@..@@@....@@@...@@@@@.@.@@@@.@.@.@@@@...@@..@@..@@@@@@..@@.@@.@@.@@.@@@.@..\n@@@...@.@@@@@.@@..@.@.@@@@@@@@.@@.@.@.@@..@@..@@@@@@@@@@.@@@@..@@.@@@@@@@@@.@.@@....@@@@.@@@@@.@@@..@@@@@@@@..@@@@@@@@@.@@..@.@@@@..@...@\n@@@@@@@@.@@@@@@@@@@@@@@....@..@@.@.@@@.@@@@@@@@@@.@@.@@@@@@@@.@....@..@@.@@@.@...@@@@.@@@@@@.@@@@..@@@@.@@..@.@@.@@@@.@.@@@..@@@@@@@@@@.@\n...@@..@.@@@@@@.@@@..@.@@.@@..@@..@.@@@.@.@.@@@@@@.@@@@@@.@@@.@@@@.@@@@..@.@@@.@...@@.@....@@@.@@@@@@.@@..@@.@@@.@.@@.@.@.@@@@.@.@@.@@..@") -> (s? t:f=w15:string)
  n2 = call <vilib>:"Delimited String to 1D String Array.vi"("delimiter"="\n", "delimited string"=w15) -> ("string array"=w13:string[])  [unwired: 9 in]
  n3 = for {
    tunnel: w13 -> [w23] mode=indexing
    tunnel: [w19] -> w9 mode=indexing
    w20 = "." ("delimiter")
    n4 = String Length(string=w23) -> (length=w22:i32)
    n5 = for {
      N: w22 -> [_]
      tunnel: w23 -> [w25]
      tunnel: [w24] -> w21 mode=indexing
      i -> [w27]
      n6 = String Subset(string=w25, offset (0)=w27, length (rest)=1 ("length (rest)")) -> (substring=w24:string)
    }
    n7 = Build Array (concatenate)(w20, w21, w20) -> (w19:string[])
  }
  n8 = Matrix Size(0:w9) -> (2:w12:i32)  [unwired: 1 out]
  n9 = Initialize Array("." ("delimiter"), w12) -> (w10:string[])
  n10 = Build Array (concatenate)(w10, w9, w10) -> (w8:string[][])
  "appended array" <- w8
  n11 = Array Size(array=w8) -> (size(s)=w7:i32[])
  "size(s)" <- w7
  n12 = Index Array(array=w7) -> (element #1=w6:i32, element #2=w5:i32)  [unwired: 2 in]
  n13 = for {
    N: 1000 -> [_]
    tunnel: w6 -> [w33]
    tunnel: w5 -> [w32]
    tunnel: [w31] -> w3 mode=concatenating
    shift-right: [w30] -> w2
    shift-left: w8 -> [w34]
    n14 = Decrement(x=w33) -> (x-1=w29:i32)
    n15 = Decrement(x=w32) -> (x-1=w28:i32)
    n16 = for {
      N: w29 -> [_]
      tunnel: w28 -> [w37]
      tunnel: [w36] -> w31 mode=indexing
      shift-right: [w35] -> w30
      shift-left: w34 -> [w39]
      i -> [w38]
      n17 = for {
        N: w37 -> [_]
        tunnel: w38 -> [w41]
        tunnel: [w44] -> w36 mode=indexing
        shift-right: [w42] -> w35
        shift-left: w39 -> [w43]
        i -> [w40]
        w50 = 1 ("index (row)")
        w51 = 3 ("length")
        n18 = Array Subset(array=w43, index (row)=w41, length (row)=w51, index (col)=w40, length (col)=w51) -> (w46:string[][])
        "subarray" <- w46
        n19 = Index Array(array=w46, index (row)=w50, index (col)=w50) -> (element=w48:string)
        n20 = Equal?(x=w48, y="@") -> (x = y?=w47:bool)
        n21 = case shown="True" w47 {
          tunnel: w46 -> [_ w84]
          tunnel: [FALSE w56] -> w45
          tunnel: w43 -> [w52 w59]
          tunnel: [w52 w60] -> w42
          tunnel: w41 -> [_ w58]
          tunnel: w40 -> [_ w57]
          frame False {
          }
          frame True {
            w81 = 2 ("index (row)")
            w82 = 1 ("index (row)")
            w83 = 0 ("index (row)")
            n22 = Increment(x=w57) -> (x+1=w54:i32)
            n23 = Index Array(array=w84, index (row) #1=w83, index (col) #1=0 ("index (col)"), index (row) #2=w83, index (col) #2=1 ("index (col)"), index (row) #3=w83, index (col) #3=2 ("index (col)"), index (row) #4=w82, index (col) #4=0 ("index (col)"), index (row) #5=w82, index (col) #5=2 ("index (col)"), index (row) #6=w81, index (col) #6=0 ("index (col)"), index (row) #7=w81, index (col) #7=1 ("index (col)"), index (row) #8=w81, index (col) #8=2 ("index (col)")) -> (element #1=w72:string, element #2=w71:string, element #3=w70:string, element #4=w69:string, element #5=w68:string, element #6=w67:string, element #7=w66:string, element #8=w65:string)
            n24 = Increment(x=w58) -> (x+1=w55:i32)
            n25 = Build Array(w72, w71, w70, w69, w68, w67, w66, w65) -> (w64:string[])
            n26 = for {
              tunnel: w64 -> [w94] mode=indexing
              tunnel: [w92] -> w61 mode=indexing
              n27 = Equal?(x=w94, y="@") -> (x = y?=w93:bool)
              n28 = Boolean To (0,1)(Boolean=w93) -> (0, 1=w92:i16)
            }
            "Array 2" <- w61
            n29 = Add Array Elements(numeric array=w61) -> (sum=w63:i16)
            n30 = Less?(x=w63, y=i16 4) -> (x < y?=w56:bool)
            "x < y?" <- w56
            n31 = case shown="True" w56 {
              tunnel: [w85 w90] -> w60
              tunnel: w59 -> [w85 w89]
              tunnel: w55 -> [_ w88]
              tunnel: w54 -> [_ w87]
              frame False {
              }
              frame True {
                n32 = Replace Array Subset(array=w89, new element="." ("new element/subarray"), index (row)=w88, index (col)=w87) -> (w90:string[][])
              }
            }
            "Array" <- w84
          }
        }
        n33 = Boolean To (0,1)(Boolean=w45) -> (0, 1=w44:i16)
      }
    }
  }
  "Array 3" <- w3
  "Array 4" <- w2
  n34 = Add Array Elements(numeric array=w3) -> (sum=→"sum":i16)
